vi "AlGaAs_Layer_V00.vi"(0 "Aluminum Flow":dbl, 1 "Al Run":bool, 2 "fDilution":dbl, 3 "Ga flow (0-10 sccm)":dbl, 4 "Ga Run":bool) -> ()   [LabVIEW 2011]
panel:
  in  "run Ga 2":bool=TRUE caption="run Ga"
  in  "run Al 2":bool caption="run Al"
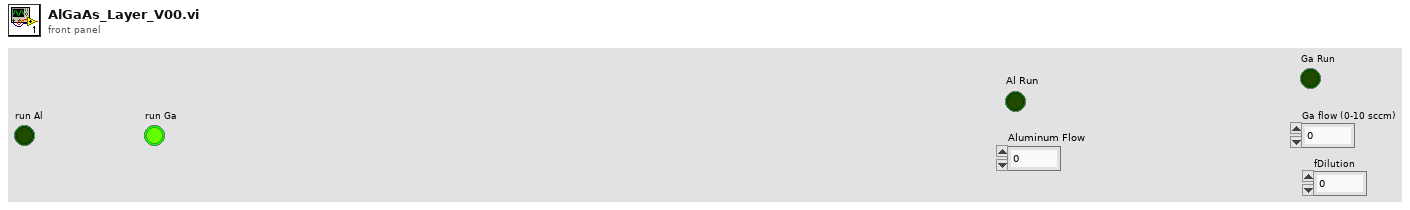
[diagram p1: front panel]
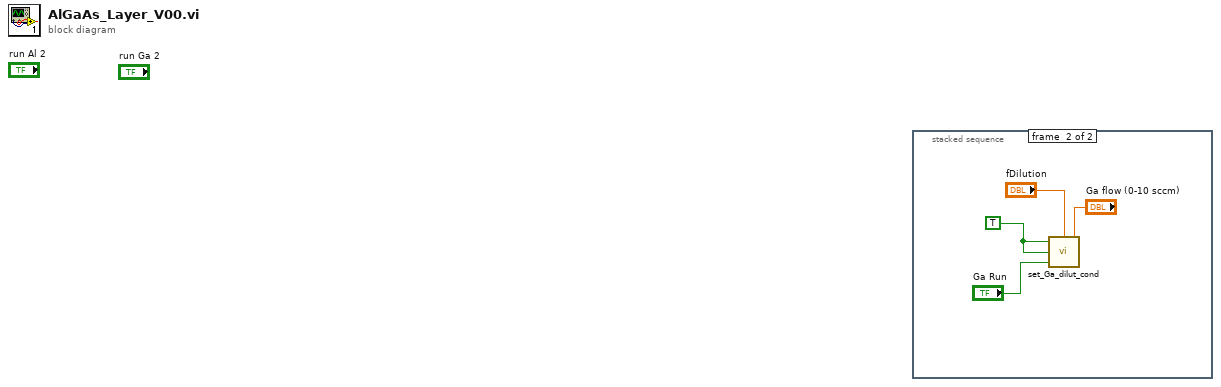
[diagram p0: block diagram]
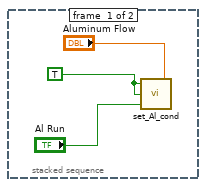
[diagram p2: hidden frame]
diagram:
  n1 = stacked-sequence {
    frame #0 {
      w3 = TRUE ("Al Active")
      n2 = call "set_Al_cond.vi"("Aluminum Flow"="Aluminum Flow", "Al Run"="Al Run", "Al Bubbler"=w3, "Al Active"=w3) -> ()
    }
    frame #1 {
      w6 = TRUE ("Active")
      n3 = call "set_Ga_dilut_cond.vi"("Ga flow (0-10 sccm)"="Ga flow (0-10 sccm)", "fDilution"="fDilution", "Run"="Ga Run", "Bubbler In"=w6, "Active"=w6) -> ()
    }
  }
